vi "Write Message Size.vi"(8 "error in (no error)":errorcluster, 10 "Message Size":T1={"Message Height"=-1, "Message Width"=-1, "Message Location"=enum."Bottom"} {"Message Width" min=-1 step=1; "Message Height" min=-1 step=1}, 11 "Popup in":refnum<class "Popup.lvclass">) -> (0 "error out":errorcluster, 3 "Popup out":refnum<class "Popup.lvclass">)   [LabVIEW 2021, in "Pop-Up.lvlib" / "Popup.lvclass"]
doc: "Write the size of the message\n\n<b>Code Developed By:</b>\nTechnology Service Corporation\n1983 S Liberty Drive\nBloomington, IN 47403\nPhone: 812 558-7100\nwww.tsc.com/atcs\n\nDeveloper:\nDaniel Coons"
uses:
  Popup.lvclass
  message info--typedef.ctl
  Popup.lvclass/Popup.ctl
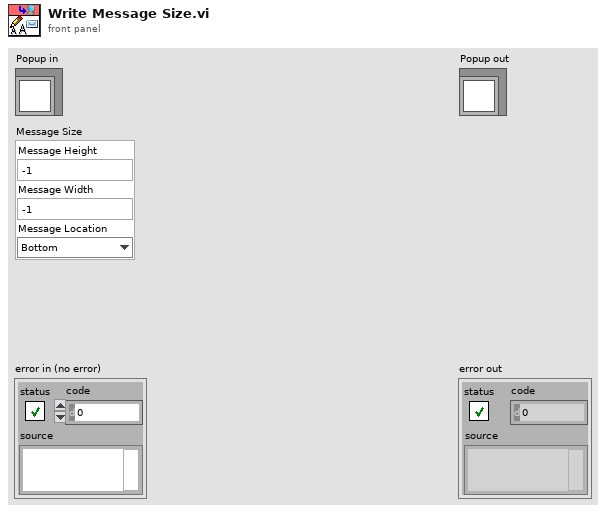
[diagram p1: front panel]
types:
  T1 = typedef "Pop-Up.lvlib/Popup.lvclass/message info--typedef.ctl" = cluster{"Message Height":i32, "Message Width":i32, "Message Location":enum16{"Top", "Bottom", "Right", "Left"}}
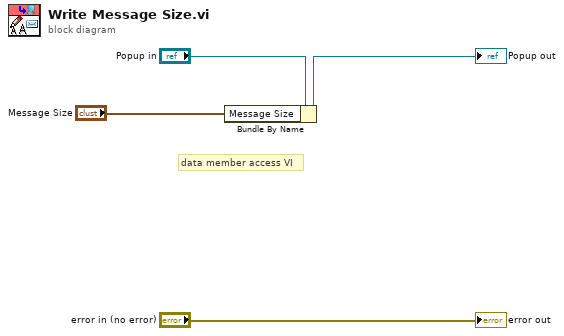
[diagram p0: block diagram]
diagram:
  # "data member access VI"
  n1 = Bundle By Name(cluster="Popup in", "Message Size"="Message Size") -> (→"Popup out":refnum<class "Popup.lvclass">)
  "error out" <- "error in (no error)"
